vi "Close.vi"(8 "error in":errorcluster, 11 "socket":refnum<class "Socket.lvclass">) -> (0 "error out":errorcluster)   [LabVIEW 2025, in "ZeroMQ.lvlib" / "Socket.lvclass"]
doc: "Signal that the socket is no longer required and to free it once pending operations are finished.\n\nNote that this is a <b>non-blocking</b> function and the socket is not necessarily closed when it returns. Any operations pending will be completed before the socket is closed and port freed. To interrupt blocking calls use ctx_destroy.\n\nDetailed API documentation: http://api.zeromq.org/3-2:zmq-close"
uses:
  Socket.lvclass
  Socket.lvclass/Socket.ctl
  libzmq-v143-mt-4_3_6/LibZMQ.lvlib
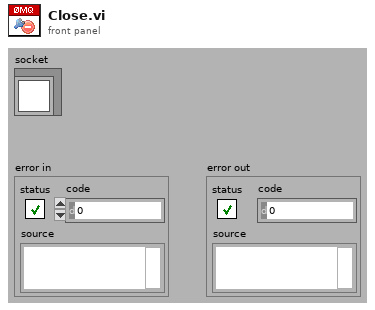
[diagram p1: front panel]
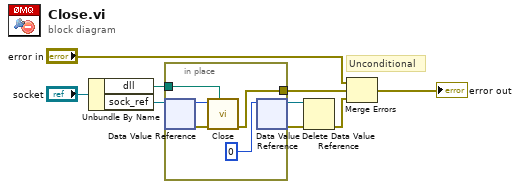
[diagram p0: block diagram]
diagram:
  # "Unconditional"
  n1 = Unbundle By Name("socket") -> ("dll"=w1:path, "sock_ref"=w8:refnum<data-value>)
  n2 = in-place {
    in-place-border: [w11] -> w4
    in-place-border: w1 -> [w10]
    n3 = in-place-dvr #1(w8) -> (w13:u64, w12:errorcluster)
    n4 = call "Close.vi"("path override"=w10, "error in (no error)"=w12, "s_"=w13) -> ("error out"=w11:errorcluster)  [unwired: 8 in]
    n5 = in-place-dvr #1(u64 0 ("data value")) -> (w6:refnum<data-value>, w7:errorcluster)
  }
  n6 = Delete Data Value Reference(data value reference=w6, error in=w7) -> (error out=w2:errorcluster)  [unwired: 1 out]
  n7 = Merge Errors("error in", w4, w2) -> (→"error out":errorcluster)
